vi "Test gRPC Timing.vi"() -> ()   [LabVIEW 2021]
uses:
  gRPC/test_service_server/test_service_server.lvlib
panel:
  in  "address":string="localhost:50051"
  in  "Run Server?":bool=TRUE
  in  "Number of Concurrent Calls (4)":i32=4
  in  "Time to Run (seconds)":i32=120
  in  "Period (msec)":i64=10
  in  "stop":bool
  in  "Run Timing Test":bool
  # "<<< Note that this\ndoesn't shut down\nthe gRPC server which\nhas its own stop button"
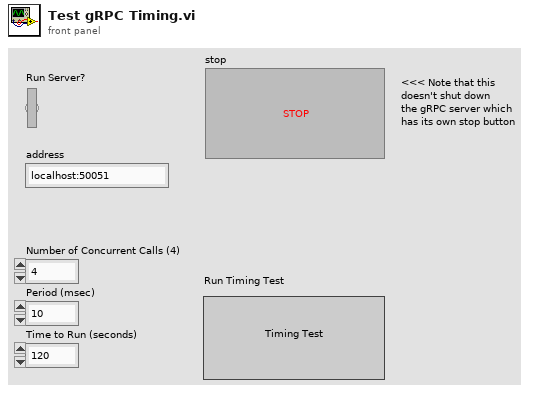
[diagram p1: front panel]
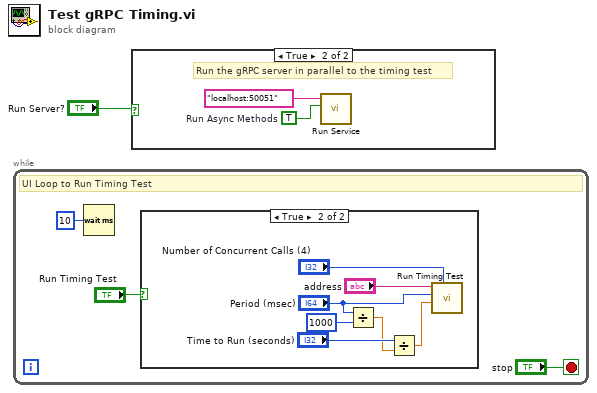
[diagram p0: block diagram]
diagram:
  n1 = while {
    stop <- "stop" stop-if-true
    # "UI Loop to Run Timing Test"
    n2 = Wait (ms)(milliseconds to wait=u32 10) -> ()  [unwired: 1 out]
    n3 = case shown="True" "Run Timing Test" {
      frame False {
      }
      frame True {
        n4 = Divide(x="Period (msec)", y=i64 1000) -> (x/y=w6:dbl)
        n5 = Divide(x="Time to Run (seconds)", y=w6) -> (x/y=w9:dbl)
        n6 = call "Run Timing Test.vi"("Number of Concurrent Calls (4)"="Number of Concurrent Calls (4)", "Number of Iterations (12000)"=w9, "Period (msec)"="Period (msec)", "address"="address") -> ()  [unwired: 5 in, 3 out]
      }
    }
  }
  n7 = case shown="True" "Run Server?" {
    frame False {
    }
    frame True {
      w13 = TRUE  # Run Async Methods
      # "Run the gRPC server in parallel to the timing test"
      n8 = call "Run Service.vi"("Async [T] / Sync [F]"=w13, "Server Address"="localhost:50051") -> ()  [unwired: 10 in]
    }
  }
